vi "GraphAsChart.vi"() -> ()   [LabVIEW 2017]
panel:
  out "Waveform Graph":dbl[][](graph)
  out "random num":dbl
  out "average":dbl
  in  "stop":bool
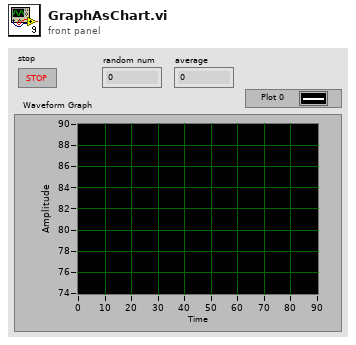
[diagram p1: front panel]
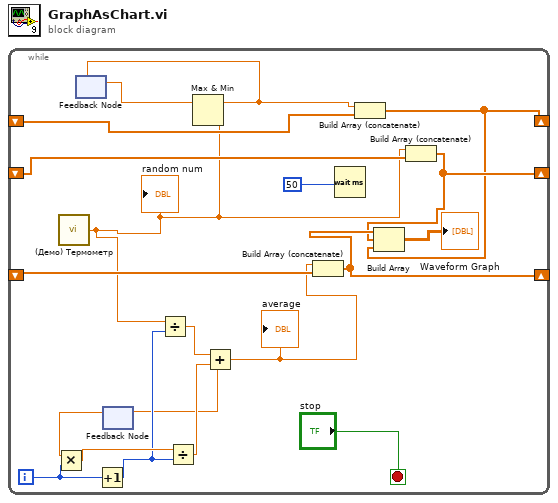
[diagram p0: block diagram]
diagram:
  n1 = while {
    shift-right: [w8] -> _
    shift-left: _ -> [w10]
    shift-right: [w4] -> _
    shift-left: _ -> [w7]
    shift-right: [w5] -> _
    shift-left: _ -> [w6]
    i -> [w16]
    stop <- "stop" stop-if-true
    n2 = call "(Демо) Термометр.vi"() -> ("Температура"=w2:dbl)  [unwired: 1 in]
    "random num" <- w2
    n3 = feedback #1() -> (w11:dbl)  [unwired: 1 in]
    n4 = Increment(x=w16) -> (x+1=w12:i32)
    n5 = feedback #2() -> (w17:dbl)  [unwired: 1 in]
    n6 = Multiply(x=w17, y=w16) -> (x*y=w15:dbl)
    n7 = Divide(x=w2, y=w12) -> (x/y=w18:dbl)
    n8 = Divide(x=w15, y=w12) -> (x/y=w13:dbl)
    n9 = Max & Min(x=w11, y=w2) -> (max(x,y)=w3:dbl)  [unwired: 1 out]
    n10 = feedback-in #1(w3) -> ()
    n11 = Add(x=w18, y=w13) -> (x+y=w1:dbl)
    "average" <- w1
    n12 = feedback-in #2(w1) -> ()
    n13 = Build Array (concatenate)(w1, w10) -> (w8:dbl[])
    n14 = Wait (ms)(milliseconds to wait=50) -> ()  [unwired: 1 out]
    n15 = Build Array (concatenate)(w3, w7) -> (w4:dbl[])
    n16 = Build Array (concatenate)(w2, w6) -> (w5:dbl[])
    n17 = Build Array(w8, w5, w4) -> (→"Waveform Graph":dbl[][])
  }
